vi "stage globals.vi"() -> ()   [LabVIEW 2016]
uses:
  Stage/Move stage command.ctl
panel:
  out "z kludge factor":ext=1.0 format="%_5g"
  out "y kludge factor":ext=1.0 format="%_5g"
  out "x kludge factor":ext=1.0 format="%_5g"
  out "Stage Handle":i32
  in  "Stage name":string="Mad City Labs 200 x 200 x 200 um USB controller"
  in  "x max (um)":ext=200.0
  out "Current Z (um)":ext=50.0 format="%_5g"
  out "Current Y (um)":ext=50.0 format="%_5g"
  out "Current X (um)":ext=50.0 format="%_5g"
  in  "Default\nstage settle time (ms)":u32=2000
  in  "Number of field steps":i16
  in  "Field step":i16
  in  "z max (um)":ext=200.0
  in  "y max (um)":ext=200.0
  out "user event out":refnum<user-event>
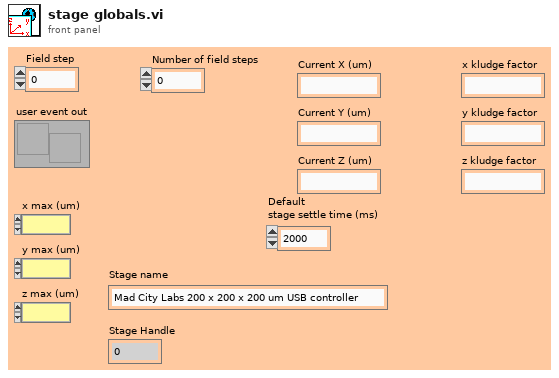
[diagram p1: front panel]
diagram:
